vi "Check Num of PTR Between Different Tester.vi"(8 "Error in":errorcluster, 11 "# of PTR":i32[](array[numeric])) -> (0 "Error out":errorcluster, 3 "Num of PTR":i32)   [LabVIEW 2018, in "STDF File Parser.lvclass"]
uses:
  STDF File Parser.lvclass
  <vilib>/Utility/error.llb/Error Cluster From Error Code.vi
  <vilib>/ErrorRing/Error Ring.xnode
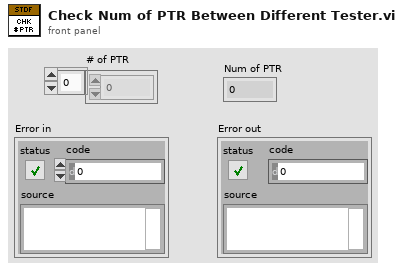
[diagram p1: front panel]
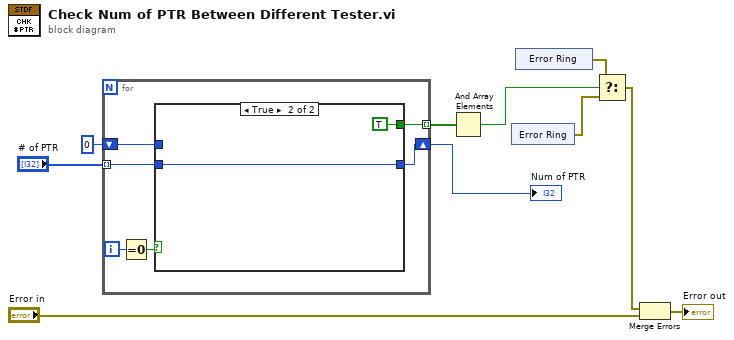
[diagram p0: block diagram]
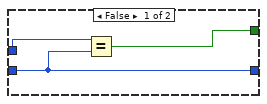
[diagram p2: hidden frame]
diagram:
  n1 = for {
    tunnel: "# of PTR" -> [w14] mode=indexing
    shift-right: [w13] -> w4
    shift-left: 0 ("Numeric") -> [w12]
    tunnel: [w11] -> w8 mode=indexing
    i -> [w16]
    n2 = Equal To 0?(x=w16) -> (x = 0?=w15:bool)
    n3 = case shown="True" w15 {
      tunnel: w14 -> [w18 w21]
      tunnel: [w18 w21] -> w13
      tunnel: w12 -> [w19 _]
      tunnel: [w17 TRUE] -> w11
      frame False {
        n4 = Equal?(x=w19, y=w18) -> (x = y?=w17:bool)
      }
      frame True {
      }
    }
  }
  "Num of PTR" <- w4
  n5 = And Array Elements(Boolean array=w8) -> (logical AND=w7:bool)
  n6 = xnode "Error Ring"() -> ("error out"=w5:errorcluster)
  n7 = xnode "Error Ring"() -> ("error out"=w6:errorcluster)
  n8 = Select(t=w6, s=w7, f=w5) -> (s? t:f=w3:errorcluster)
  n9 = Merge Errors(w3, "Error in") -> (→"Error out":errorcluster)
